vi "Dynamic call-Time series editor.vi"(8 "error in (no error)":errorcluster) -> (0 "error out":errorcluster)   [LabVIEW 2020]
uses:
  Visualisation/Timelapse Viewer/Globals/gl_Time series viewer globals.vi
panel:
  out "Window is open":bool
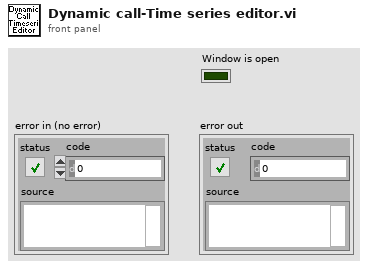
[diagram p1: front panel]
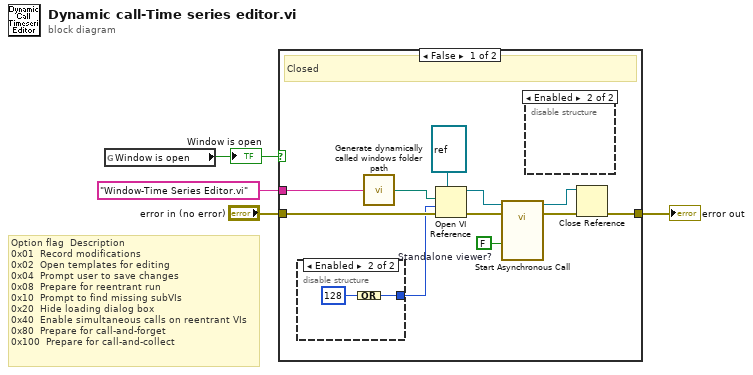
[diagram p0: block diagram]
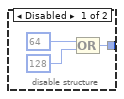
[diagram p2: hidden frame]
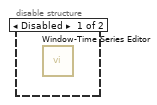
[diagram p3: hidden frame]
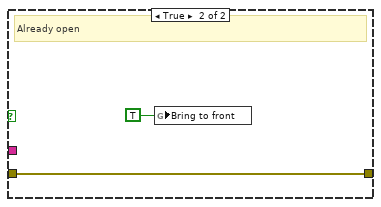
[diagram p4: hidden frame]
diagram:
  # "Option flag \tDescription\n0x01 \tRecord modifications\n0x02 \tOpen templates for editing\n0x04 \tPrompt user to save changes\n0x08 \tPrepare for reentrant run\n0x10 \tPrompt to find missing subVIs\n0x20 \tHide loading dialog box\n0x40 \tEnable simultaneous calls on reentrant VIs\n0x80 \tPrepare for call-and-forget\n0x100 \tPrepare for call-and-collect"
  n1 = global read "gl_Time series viewer globals.vi" "Window is open"() -> (w1:bool)
  "Window is open" <- w1
  n2 = case shown="False" w1 {
    tunnel: "error in (no error)" -> [w15 w21]
    tunnel: [w14 w21] -> w3
    tunnel: "Window-Time Series Editor.vi" ("Error Source") -> [w12 _]
    frame False {
      w5 = FALSE  # Standalone viewer?
      # "Closed"
      n3 = disable-structure shown="Enabled" {
        disable-tunnel: [w18 w20] -> w9
        frame Disabled {
          n4 = Compound Arithmetic op=OR(64, 128) -> (w18:i32)
        }
        frame Enabled {
          n5 = Compound Arithmetic op=OR(128) -> (w20:i32)
        }
      }
      n6 = call "Generate dynamically called windows folder path.vi"("name of dynamically called VI"=w12) -> ("Dynamically called VI path"=w13:path)
      n7 = Open VI Reference(type specifier VI Refnum (for type only)=refnum<vi> refnum, vi path=w13, options=w9, error in (no error)=w15) -> (vi reference=w10:refnum<vi>, error out=w11:errorcluster)  [unwired: 2 in]
      n8 = call-by-ref "Start Asynchronous Call"(reference=w10, error in=w11, "Standalone viewer?"=w5) -> (reference out=w6:refnum<vi>, error out=w7:errorcluster)  [unwired: 11 in]
      n9 = disable-structure shown="Enabled" {
        frame Disabled {
          n10 = call "Window-Time Series Editor.vi"() -> ()  [unwired: 12 in]
        }
        frame Enabled {
        }
      }
      n11 = Close Reference(reference=w6, error in (no error)=w7) -> (error out=w14:errorcluster)
    }
    frame True {
      # "Already open"
      n12 = global write "gl_Time series viewer globals.vi" "Bring to front"(TRUE ("Bring Timelapse Editor to front")) -> ()
    }
  }
  "error out" <- w3
